vi "UEvent_MEASURE_SEQ3_DAQ.vi"(8 "error in (no error)":errorcluster, 10 "USB in":tag, 11 "Range - Shunts":T1) -> (0 "error out":errorcluster, 1 "DUT_Voltage":dbl, 2 "Battery_Voltage":dbl, 3 "Refnum out":refnum<k21>)   [LabVIEW 2015]
uses:
  Range_Shunt_selector.ctl
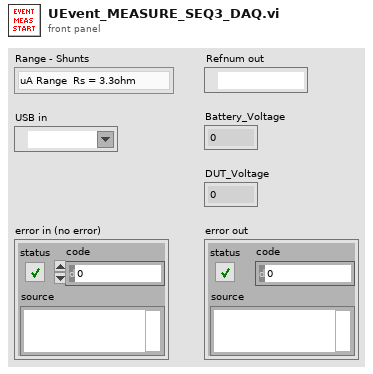
[diagram p1: front panel]
types:
  T1 = typedef "Range_Shunt_selector.ctl" = enum16{"uA Range  Rs = 3.3ohm", "mA Range Rs = 3.3ohm", "mA Range Rs = 1ohm", "mA Range Rs = 1ohm - X2"}
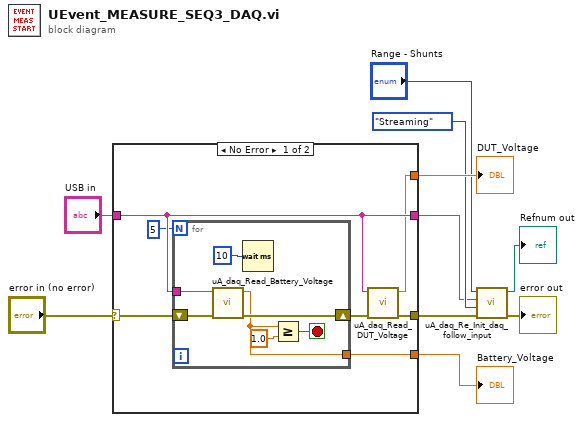
[diagram p0: block diagram]
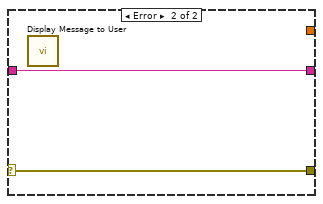
[diagram p2: hidden frame]
diagram:
  n1 = case shown="No Error" "error in (no error)" {
    selector: "error in (no error)" -> [w16 w26]
    tunnel: "USB in" -> [w14 w25]
    tunnel: [w15 w26] -> w6
    tunnel: [w14 w25] -> w4
    tunnel: [w11 _] -> w9
    tunnel: [w13 _] -> w10
    frame No Error {
      n2 = for {
        N: 5 -> [_]
        tunnel: w14 -> [w22]
        shift-right: [w24] -> w17
        shift-left: w16 -> [w23]
        tunnel: [w20] -> w11
        stop <- w21 stop-if-true
        n3 = call "uA_daq_Read_Battery_Voltage.vi"("error in"=w23, "USB DAQ"=w22) -> ("error out"=w24:errorcluster, "Battery_Voltage"=w20:dbl)  [unwired: 8 in]
        n4 = Wait (ms)(milliseconds to wait=u32 10) -> ()  [unwired: 1 out]
        n5 = Greater Or Equal?(x=w20, y=1.0) -> (x >= y?=w21:bool)
      }
      n6 = call "uA_daq_Read_DUT_Voltage.vi"("error in"=w17, "USB DAQ"=w14) -> ("error out"=w15:errorcluster, "DUT_Voltage"=w13:dbl)  [unwired: 8 in]
    }
    frame Error {
      n7 = call "Display Message to User"() -> ()  [unwired: 10 in, 2 out]
    }
  }
  "DUT_Voltage" <- w10
  "Battery_Voltage" <- w9
  n8 = call "uA_daq_Re_Init_daq_follow_input.vi"("error in (no error)"=w6, "Acquire Mode"=enum16{"Streaming", "Read All", "Stop"}."Streaming", "USB"=w4, "Range_shunt"="Range - Shunts") -> ("error out"=→"error out":errorcluster, "Refnum out"=→"Refnum out":refnum<k21>)  [unwired: 6 in]
